vi "Test Data to Wave.vi"() -> ()   [LabVIEW 2019]
uses:
  <vilib>/addons/_JKI Toolkits/Caraya/classes/Test/Test.lvclass
panel:
  out "error out":errorcluster
  in  "8 bit integer":i8
  in  "16 bit integer":i16
  in  "32 bit integer":i32
  in  "single precision float":sgl
  in  "double precision float":dbl format="%#_13g"
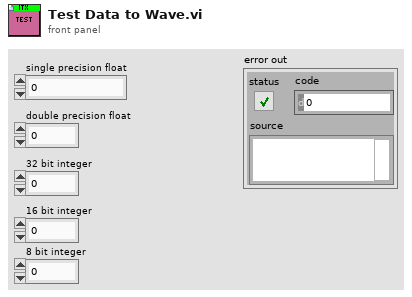
[diagram p1: front panel]
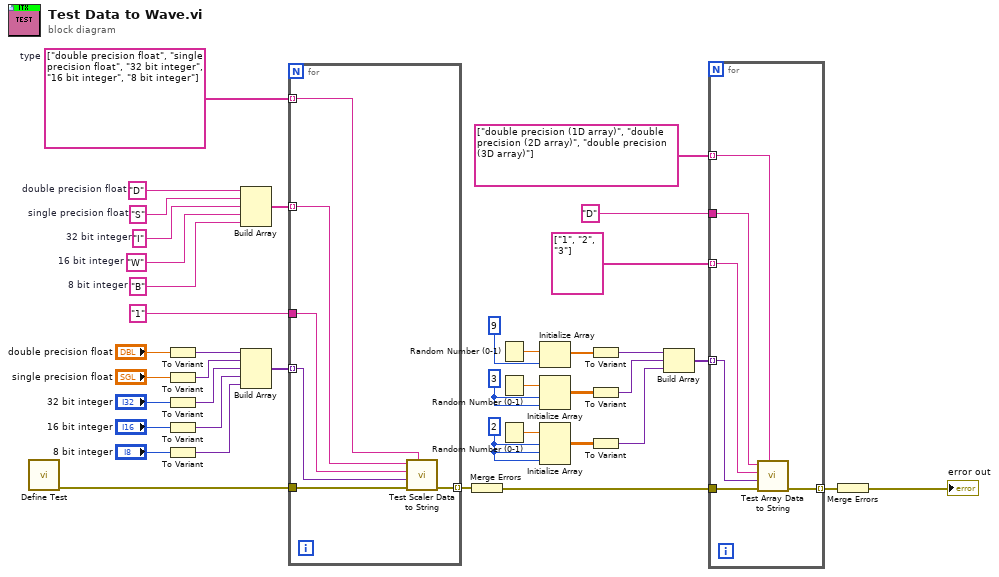
[diagram p0: block diagram]
diagram:
  w2 = 2
  w3 = 3
  w20 = string[] ["double precision float", "single precision float", "32 bit integer", "16 bit integer", "8 bit integer"]  # type
  w28 = "B"  # 8 bit integer
  w29 = "W"  # 16 bit integer
  w30 = "I"  # 32 bit integer
  w24 = "S"  # single precision float
  w23 = "D"  # double precision float
  n1 = call <vilib>:"Define Test.vi"() -> ("error out"=w39:errorcluster)  [unwired: 10 in, 1 out]
  n2 = To Variant(anything="double precision float") -> (Variant=w35:variant)
  n3 = To Variant(anything="single precision float") -> (Variant=w34:variant)
  n4 = To Variant(anything="32 bit integer") -> (Variant=w33:variant)
  n5 = To Variant(anything="16 bit integer") -> (Variant=w32:variant)
  n6 = To Variant(anything="8 bit integer") -> (Variant=w31:variant)
  n7 = Build Array(w23, w24, w30, w29, w28) -> (w27:string[])
  n8 = Build Array(w35, w34, w33, w32, w31) -> (w26:variant[])
  n9 = for {
    tunnel: "1" ("Label") -> [w46]
    tunnel: w27 -> [w45] mode=indexing
    tunnel: w39 -> [w43]
    tunnel: w26 -> [w42] mode=indexing
    tunnel: [w44] -> w25 mode=indexing
    tunnel: w20 -> [w41] mode=indexing
    n10 = call "Test Scaler Data to String.vi"("Datatype"=w41, "error in (no error)"=w43, "Data"=w42, "Dimension"=w46, "Flag"=w45) -> ("error out"=w44:errorcluster)  [unwired: 6 in]
  }
  n11 = Merge Errors(w25) -> (w19:errorcluster)
  n12 = Random Number (0-1)() -> (number: 0 to 1=w16:dbl)
  n13 = Random Number (0-1)() -> (number: 0 to 1=w17:dbl)
  n14 = Random Number (0-1)() -> (number: 0 to 1=w18:dbl)
  n15 = Initialize Array(w16, 9) -> (w12:dbl[])
  n16 = Initialize Array(w17, w3, w3) -> (w11:dbl[][])
  n17 = Initialize Array(w18, w2, w2, w2) -> (w10:dbl[][][])
  n18 = To Variant(anything=w12) -> (Variant=w13:variant)
  n19 = To Variant(anything=w11) -> (Variant=w14:variant)
  n20 = To Variant(anything=w10) -> (Variant=w9:variant)
  n21 = Build Array(w13, w14, w9) -> (w8:variant[])
  n22 = for {
    tunnel: string[] ["double precision (1D array)", "double precision (2D array)", "double precision (3D array)"] ("Datatype") -> [w52] mode=indexing
    tunnel: w8 -> [w49] mode=indexing
    tunnel: string[] ["1", "2", "3"] ("Label") -> [w48] mode=indexing
    tunnel: "D" ("Flag") -> [w47]
    tunnel: w19 -> [w51]
    tunnel: [w50] -> w4 mode=indexing
    n23 = call "Test Array Data to String.vi"("Datatype"=w52, "error in (no error)"=w51, "Data"=w49, "Dimension"=w48, "Flag"=w47) -> ("error out"=w50:errorcluster)  [unwired: 6 in]
  }
  n24 = Merge Errors(w4) -> (→"error out":errorcluster)
